vi "pivot_right_state.vi"(0 "state in":T1={"State"=enum."sense", "Maze"=[[FALSE, FALSE, FALSE, FALSE, FALSE, FALSE, FALSE, FALSE, FALSE], [FALSE, FALSE, TRUE, FALSE, FALSE, TRUE, TRUE, TRUE, FALSE], [FALSE, FALSE, TRUE, TRUE, TRUE, TRUE, FALSE, FALSE, FALSE], [FALSE, FALSE, TRUE, FALSE, FALSE, TRUE, FALSE, FALSE, FALSE], [TRUE, TRUE, TRUE, FALSE, FALSE, TRUE, FALSE, TRUE, TRUE], [FALSE, FALSE, FALSE, TRUE, TRUE, TRUE, FALSE, TRUE, FALSE], [FALSE, FALSE, FALSE, FALSE, FALSE, TRUE, TRUE, TRUE, FALSE], [FALSE, FALSE, FALSE, FALSE, FALSE, FALSE, FALSE, FALSE, FALSE], [FALSE, FALSE, FALSE, FALSE, FALSE, FALSE, FALSE, FALSE, FALSE]], "Runner Row"=0, "Runner Column"=0, "Runner Direction"=enum."east", "Sense"={"wall in front"=FALSE, "wall to left"=FALSE, "wall to right"=FALSE, "wall behind"=FALSE, "exit column"=FALSE}, "Hand"=enum."Left-handed"}) -> (4 "state out":T1={"State"=enum."sense", "Maze"=[[FALSE, FALSE, FALSE, FALSE, FALSE, FALSE, FALSE, FALSE, FALSE], [FALSE, FALSE, TRUE, FALSE, FALSE, TRUE, TRUE, TRUE, FALSE], [FALSE, FALSE, TRUE, TRUE, TRUE, TRUE, FALSE, FALSE, FALSE], [FALSE, FALSE, TRUE, FALSE, FALSE, TRUE, FALSE, FALSE, FALSE], [TRUE, TRUE, TRUE, FALSE, FALSE, TRUE, FALSE, TRUE, TRUE], [FALSE, FALSE, FALSE, TRUE, TRUE, TRUE, FALSE, TRUE, FALSE], [FALSE, FALSE, FALSE, FALSE, FALSE, TRUE, TRUE, TRUE, FALSE], [FALSE, FALSE, FALSE, FALSE, FALSE, FALSE, FALSE, FALSE, FALSE], [FALSE, FALSE, FALSE, FALSE, FALSE, FALSE, FALSE, FALSE, FALSE]], "Runner Row"=0, "Runner Column"=0, "Runner Direction"=enum."east", "Sense"={"wall in front"=FALSE, "wall to left"=FALSE, "wall to right"=FALSE, "wall behind"=FALSE, "exit column"=FALSE}, "Hand"=enum."Left-handed"})   [LabVIEW 2016]
uses:
  typedefs/state.ctl
  typedefs/action_start.ctl
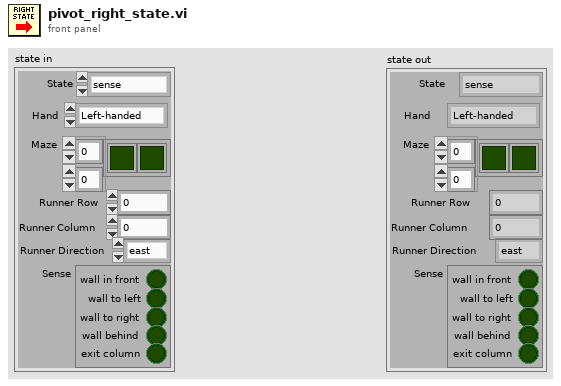
[diagram p1: front panel]
types:
  T1 = typedef "state.ctl" = cluster{"State":T2, "Maze":bool[][], "Runner Row":i32, "Runner Column":i32, "Runner Direction":enum16{"east", "north", "west", "south"}, "Sense":cluster{"wall in front":bool, "wall to left":bool, "wall to right":bool, "wall behind":bool, "exit column":bool}, "Hand":enum16{"Left-handed", "Right-handed"}}
  T2 = typedef "action_start.ctl" = enum16{"sense", "decide", "step", "pivot right", "pivot left", "stop"}
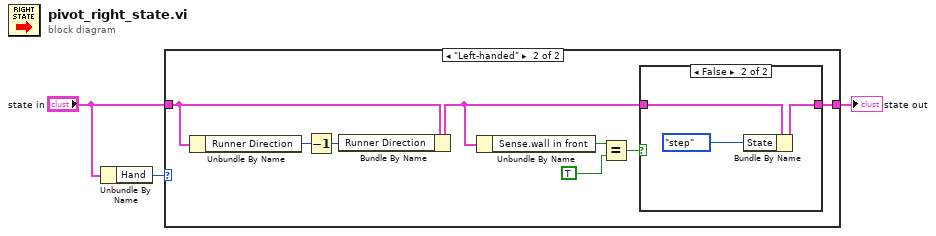
[diagram p0: block diagram]
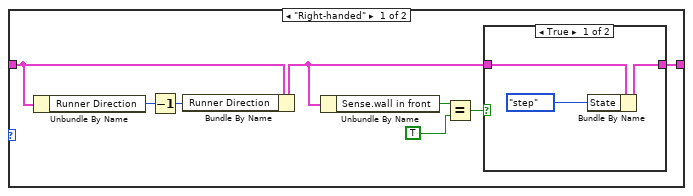
[diagram p2: hidden frame]
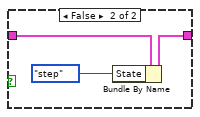
[diagram p3: hidden frame]
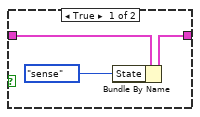
[diagram p4: hidden frame]
diagram:
  n1 = Unbundle By Name("state in") -> ("Hand"=w2:enum16{"Left-handed", "Right-handed"})
  n2 = case shown="\"Left-handed\"" w2 {
    tunnel: [w6 w20] -> w3
    tunnel: "state in" -> [w5 w19]
    frame "Right-handed" {
      n3 = Unbundle By Name(w5) -> ("Runner Direction"=w11:enum16{"east", "north", "west", "south"})
      n4 = Decrement(x=w11) -> (x-1=w10:enum16{"east", "north", "west", "south"})
      n5 = Bundle By Name(cluster=w5, "Runner Direction"=w10) -> (w4:T1)
      n6 = Unbundle By Name(w4) -> ("Sense.wall in front"=w9:bool)
      n7 = Equal?(x=w9, y=TRUE) -> (x = y?=w7:bool)
      n8 = case shown="True" w7 {
        tunnel: w4 -> [w13 w16]
        tunnel: [w12 w15] -> w6
        frame True {
          n9 = Bundle By Name(cluster=w13, "State"=action_start."step" ("action start")) -> (w12:T1)
        }
        frame False {
          n10 = Bundle By Name(cluster=w16, "State"=action_start."step" ("action start")) -> (w15:T1)
        }
      }
    }
    frame "Left-handed" {
      n11 = Unbundle By Name(w19) -> ("Runner Direction"=w25:enum16{"east", "north", "west", "south"})
      n12 = Decrement(x=w25) -> (x-1=w24:enum16{"east", "north", "west", "south"})
      n13 = Bundle By Name(cluster=w19, "Runner Direction"=w24) -> (w18:T1)
      n14 = Unbundle By Name(w18) -> ("Sense.wall in front"=w23:bool)
      n15 = Equal?(x=w23, y=TRUE) -> (x = y?=w21:bool)
      n16 = case shown="False" w21 {
        tunnel: w18 -> [w27 w30]
        tunnel: [w26 w29] -> w20
        frame True {
          n17 = Bundle By Name(cluster=w27, "State"=action_start."sense" ("action start")) -> (w26:T1)
        }
        frame False {
          n18 = Bundle By Name(cluster=w30, "State"=action_start."step" ("action start")) -> (w29:T1)
        }
      }
    }
  }
  "state out" <- w3
